vi "System-TDK-HVPS.vi"() -> ()   [LabVIEW 2016, in "DSI-RT.lvlib"]
uses:
  DSI-RT.lvlib
  <vilib>/addons/Software Calibration Management/xSCM/CalPoint.xnode
  <vilib>/addons/Software Calibration Management/xSCM/ni_scm.dll
panel:
  out "error out":errorcluster {"code" format="%.0x"}
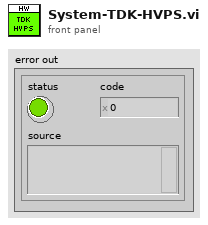
[diagram p1: front panel]
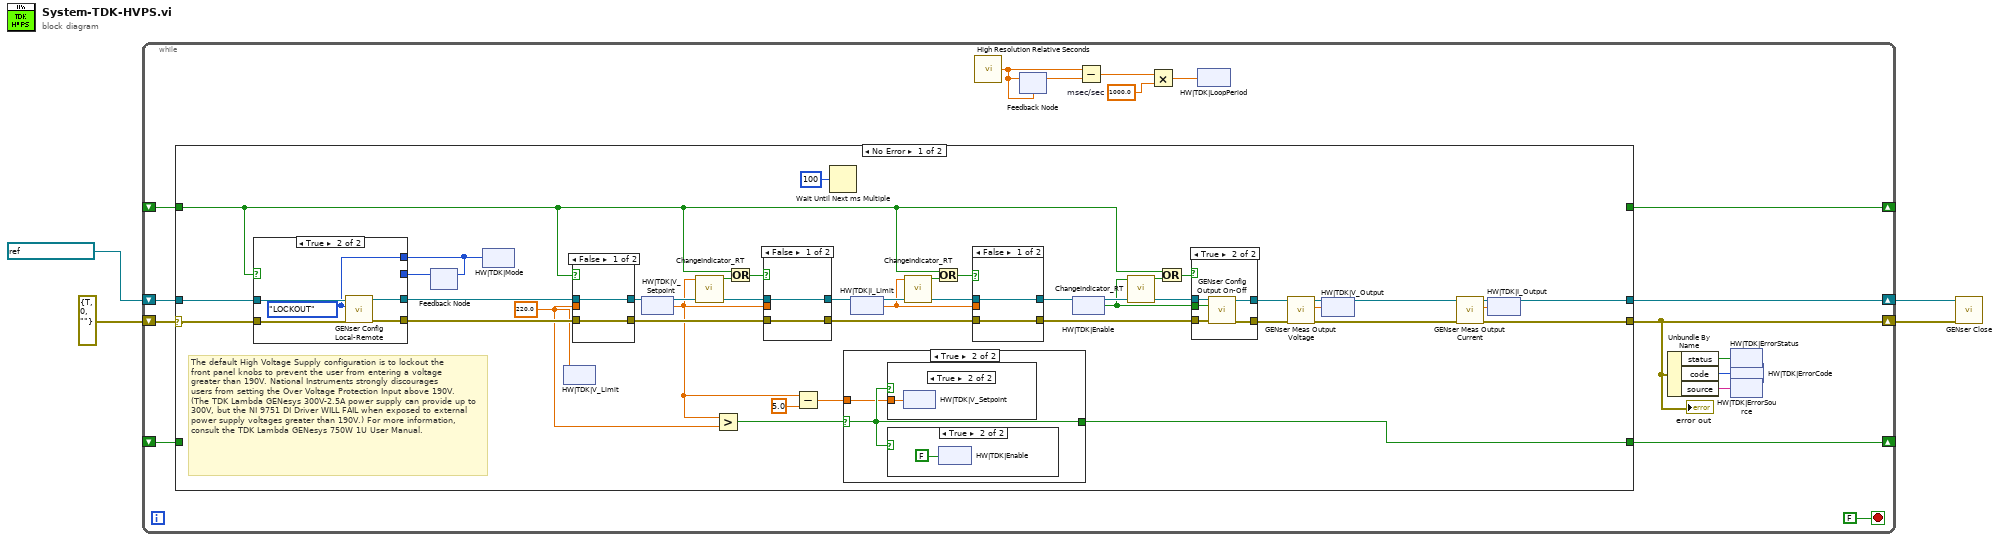
[diagram p0: block diagram]
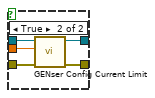
[diagram p6: hidden frame]
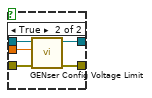
[diagram p7: hidden frame]
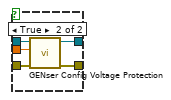
[diagram p8: hidden frame]
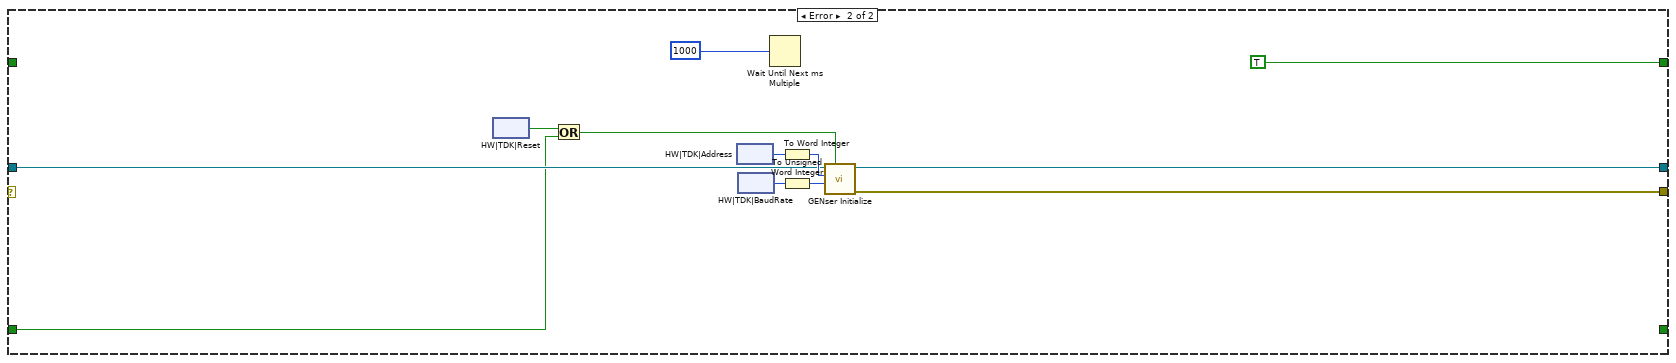
[diagram p10: hidden frame]
diagram:
  n1 = while {
    shift-right: [w15] -> w3
    shift-left: refnum<visa-resource-name> "ASRL1::INSTR" ("VISA In") -> [w17]
    shift-right: [w7] -> w2
    shift-left: errorcluster {"status"=TRUE, "code"=0, "source"=""} ("error constant") -> [w16]
    shift-right: [w14] -> _
    shift-left: _ -> [w13]
    shift-right: [w12] -> _
    shift-left: _ -> [w11]
    stop <- FALSE stop-if-true
    w5 = 1000.0  # msec/sec
    n2 = case shown="No Error" w16 {
      selector: w16 -> [w42 _]
      tunnel: [w57 w152] -> w15
      tunnel: [w43 w153] -> w7
      tunnel: w17 -> [w56 w155]
      tunnel: [_ TRUE] -> w14
      tunnel: w13 -> [w28 _]
      tunnel: [w33 _] -> w12
      tunnel: w11 -> [_ w149]
      frame No Error {
        w27 = sgl 220.0 ("Value")
        # "The default High Voltage Supply configuration is to lockout the \nfront panel knobs to prevent the user from entering a voltage \ngreater than 190V. National Instruments strongly discourages \nusers from setting the Over Voltage Protection Input above 190V. (The TDK Lambda GENesys 300V-2.5A power supply can provide up to 300V, but the NI 9751 DI Driver WILL FAIL when exposed to external power supply voltages greater than 190V.) For more information, consult the TDK Lambda GENesys 750W 1U User Manual."
        n3 = feedback #1() -> (w25:enum16{"LOCAL", "REMOTE", "LOCKOUT"})  [unwired: 1 in]
        n4 = case shown="True" w28 {
          tunnel: w56 -> [w87 w92]
          tunnel: [w86 w91] -> w47
          tunnel: [w87 w90] -> w46
          tunnel: w42 -> [w86 w89]
          tunnel: [w85 w88] -> w26
          tunnel: w25 -> [w85 _]
          frame False {
          }
          frame True {
            w88 = enum16{"LOCAL", "REMOTE", "LOCKOUT"}."LOCKOUT" ("Mode")
            n5 = call <instrlib>:"GENser Config Local-Remote.vi"("error"=w89, "Mode"=w88, "VISA"=w92) -> ("error out"=w91:errorcluster, "VISA out"=w90:refnum<visa-resource-name>)  [unwired: 7 in]
          }
        }
        n6 = feedback-in #1(w26) -> ()
        n7 = xnode "HW|TDK|Mode"("Value"=w26) -> ()
        n8 = xnode "HW|TDK|V_Limit"("Value"=w27) -> ()
        n9 = case shown="False" w28 {
          tunnel: w47 -> [w122 w128]
          tunnel: w46 -> [w123 w127]
          tunnel: [w123 w126] -> w45
          tunnel: [w122 w125] -> w44
          tunnel: w27 -> [_ w124]
          frame False {
          }
          frame True {
            n10 = call <instrlib>:"GENser Config Voltage Protection.vi"("error"=w128, "OVP Level"=w124, "VISA"=w127) -> ("error out"=w125:errorcluster, "VISA out"=w126:refnum<visa-resource-name>)  [unwired: 7 in]
          }
        }
        n11 = xnode "HW|TDK|V_Setpoint"() -> ("Value"=w30:sgl)
        n12 = call "ChangeIndicator_RT.vi"("Input"=w30) -> ("Change"=w41:bool)  [unwired: 9 in]
        n13 = Greater?(x=w30, y=w27) -> (0:w29:bool)
        n14 = Or(x=w28, y=w41) -> (x .or. y?=w40:bool)
        n15 = case shown="False" w40 {
          tunnel: [w115 w121] -> w51
          tunnel: [w116 w120] -> w50
          tunnel: w30 -> [_ w119]
          tunnel: w45 -> [w116 w118]
          tunnel: w44 -> [w115 w117]
          frame False {
          }
          frame True {
            n16 = call <instrlib>:"GENser Config Voltage Limit.vi"("error"=w117, "Volt Limit"=w119, "VISA"=w118) -> ("error out"=w121:errorcluster, "VISA out"=w120:refnum<visa-resource-name>)  [unwired: 7 in]
          }
        }
        n17 = Subtract(x=w30, y=sgl 5.0) -> (x-y=w31:sgl)
        n18 = Wait Until Next ms Multiple(millisecond multiple=u32 100) -> ()  [unwired: 1 out]
        n19 = case shown="True" w29 {
          selector: w29 -> [_ w94]
          tunnel: [_ w94] -> w33
          tunnel: w31 -> [_ w93]
          frame False {
          }
          frame True {
            n20 = case shown="True" w94 {
              tunnel: w93 -> [_ w100]
              frame False {
              }
              frame True {
                n21 = xnode "HW|TDK|V_Setpoint"("Value"=w100) -> ()
              }
            }
            n22 = case shown="True" w94 {
              frame False {
              }
              frame True {
                n23 = xnode "HW|TDK|Enable"("Value"=FALSE) -> ()
              }
            }
          }
        }
        n24 = xnode "HW|TDK|I_Limit"() -> ("Value"=w37:sgl)
        n25 = call "ChangeIndicator_RT.vi"("Input"=w37) -> ("Change"=w38:bool)  [unwired: 9 in]
        n26 = Or(x=w28, y=w38) -> (x .or. y?=w39:bool)
        n27 = case shown="False" w39 {
          tunnel: [w108 w114] -> w53
          tunnel: [w109 w113] -> w52
          tunnel: w51 -> [w108 w112]
          tunnel: w50 -> [w109 w111]
          tunnel: w37 -> [_ w110]
          frame False {
          }
          frame True {
            n28 = call <instrlib>:"GENser Config Current Limit.vi"("error"=w112, "Current Limit"=w110, "VISA"=w111) -> ("error out"=w114:errorcluster, "VISA out"=w113:refnum<visa-resource-name>)  [unwired: 7 in]
          }
        }
        n29 = xnode "HW|TDK|Enable"() -> ("Value"=w34:bool)
        n30 = call "ChangeIndicator_RT.vi"("Input"=w34) -> ("Change"=w35:bool)  [unwired: 9 in]
        n31 = Or(x=w28, y=w35) -> (x .or. y?=w36:bool)
        n32 = case shown="True" w36 {
          tunnel: w53 -> [w142 w148]
          tunnel: w52 -> [w143 w147]
          tunnel: [w143 w146] -> w49
          tunnel: [w142 w145] -> w48
          tunnel: w34 -> [_ w144]
          frame False {
          }
          frame True {
            n33 = call <instrlib>:"GENser Config Output On-Off.vi"("error"=w148, "Output ON"=w144, "VISA"=w147) -> ("error out"=w145:errorcluster, "VISA out"=w146:refnum<visa-resource-name>)  [unwired: 7 in]
          }
        }
        n34 = call <instrlib>:"GENser Meas Output Voltage.vi"("error"=w48, "VISA"=w49) -> ("error out"=w55:errorcluster, "Output Voltage"=w22:dbl, "VISA out"=w54:refnum<visa-resource-name>)  [unwired: 7 in]
        n35 = xnode "HW|TDK|V_Output"("Value"=w22) -> ()
        n36 = call <instrlib>:"GENser Meas Output Current.vi"("error"=w55, "VISA"=w54) -> ("error out"=w43:errorcluster, "Output Current"=w23:dbl, "VISA out"=w57:refnum<visa-resource-name>)  [unwired: 7 in]
        n37 = xnode "HW|TDK|I_Output"("Value"=w23) -> ()
      }
      frame Error {
        n38 = xnode "HW|TDK|Reset"() -> ("Value"=w160:bool)
        n39 = Or(x=w160, y=w149) -> (x .or. y?=w150:bool)
        n40 = xnode "HW|TDK|Address"() -> ("Value"=w157:i32)
        n41 = xnode "HW|TDK|BaudRate"() -> ("Value"=w156:enum32{"1200", "2400", "4800", "9600", "19200"})
        n42 = Wait Until Next ms Multiple(millisecond multiple=u32 1000) -> ()  [unwired: 1 out]
        n43 = To Word Integer(number=w157) -> (16bit integer=w158:i16)
        n44 = To Unsigned Word Integer(number=w156) -> (unsigned 16bit integer=w159:u16)
        n45 = call <instrlib>:"GENser Initialize.vi"("Reset (T)"=w150, "BAUD"=w159, "GEN Addr"=w158, "VISA name"=w155) -> ("error out"=w153:errorcluster, "VISA out"=w152:refnum<visa-resource-name>)  [unwired: 6 in]
      }
    }
    "error out" <- w7
    n46 = call <vilib>:"High Resolution Relative Seconds.vi"() -> ("relative seconds"=w20:dbl)
    n47 = feedback #2(w20) -> (w19:dbl)
    n48 = feedback-in #2(w20) -> ()
    n49 = Subtract(x=w20, y=w19) -> (x-y=w21:dbl)
    n50 = Multiply(x=w21, y=w5) -> (x*y=w18:dbl)
    n51 = xnode "HW|TDK|LoopPeriod"("Value"=w18) -> ()
    n52 = Unbundle By Name(w7) -> ("status"=w8:bool, "code"=w9:i32, "source"=w10:string)
    n53 = xnode "HW|TDK|ErrorStatus"("Value"=w8) -> ()
    n54 = xnode "HW|TDK|ErrorCode"("Value"=w9) -> ()
    n55 = xnode "HW|TDK|ErrorSource"("Value"=w10) -> ()
  }
  n56 = call <instrlib>:"GENser Close.vi"("error"=w2, "VISA name"=w3) -> ()  [unwired: 9 in, 1 out]
